vi "Puff_Dose.vi"() -> (5 "Plug in titles":string[](array[string]), 7 "Plug in values":string[](array[string]))   [LabVIEW 2022 SP3]
uses:
  Controls/Inst_type.ctl
  File/File Update Cluster.ctl
  Globals/Meas_global.vi
panel:
  in  "Show Puff Panel":bool=TRUE
  in  "Puff Stats only?":bool
  in  "Save Av puff files":bool=TRUE
  in  "Saved trace length":i32=200
  in  "Save individual puff files":bool
  in  "File Extension":string=".xls"
  in  "Save Puff Analysis file":bool
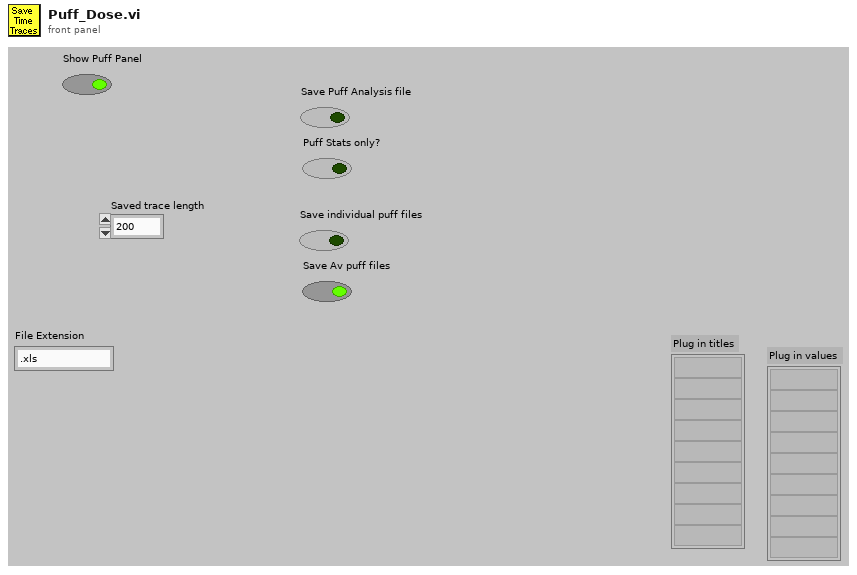
[diagram p1: front panel]
types:
  T1 = typedef "Inst_type.ctl" = enum16{"Raw voltage", "Raw with zero offsetting", "Propeller anemometer", "Pressure Transducer", "Pitot-static tube", "Hot wire", "Cross wire 1", "Cross wire 2", "Generic Linear", "Generic Polynomial", "Generic BackPoly", "Fast FID", "Thermocouple", "Cold wire", "Pulsed Wire", "LDA Vel", "LDA Tran time", "LDA Arr time", "Microphone"}
  T2 = typedef "File Update Cluster.ctl" = cluster{"File Path":path, "Rows to Add":i32[], "Extra Ch Names":string[], "Extra Ch Values":string[], "Initial Header String":string, "Separation Character":enum16{"Tab", "Comma"}}
  T3 = typedef "Analysis_info_cluster.ctl" = cluster{"Colour":u32, "Inst type":T1, "Inst name":string, "Symbol":string, "Code name":string, "Extra Info":string, "Inst Array":T4, "Extra Titles":string[], "Extra Values":string[], "U":dbl, "u^2":dbl, "u^3":dbl, "u^4":dbl, "Skew_u":dbl, "Kurt_u":dbl, "Sd Error in Mean":dbl, "% u'/U":dbl, "X":dbl, "Y":dbl, "Z":dbl, "Timescale integral Estimate":dbl, "Sd Error in Variance":dbl, "Calib File":path, "Calib Constants":dbl[], "Output Position":bool, "Stats":enum16{"None", "Basic", "Full"}, "Av Sampling Rate":dbl, "Av No of Samples":dbl, "Total Meas Time (s)":dbl, "ADAM Ch Name":string, "Max value":dbl, "Min value":dbl, "Req Sample Rate Hz":dbl, "Sync Delay Time (s)":dbl, "Ch No":i16, "Device":string, "Use Latest Calib":bool, "Port":string, "Metadata Ch Names":string[], "Metadata Ch Values":string[], "Label":string, "chState":T5, "Point Drift":dbl}
  T4 = typedef "Instrument_Array.ctl" = enum16{"PWA", "LDA", "Analogue"}
  T5 = typedef "channelState.ctl" = enum32{"No Selection", "Solo", "Mute"}
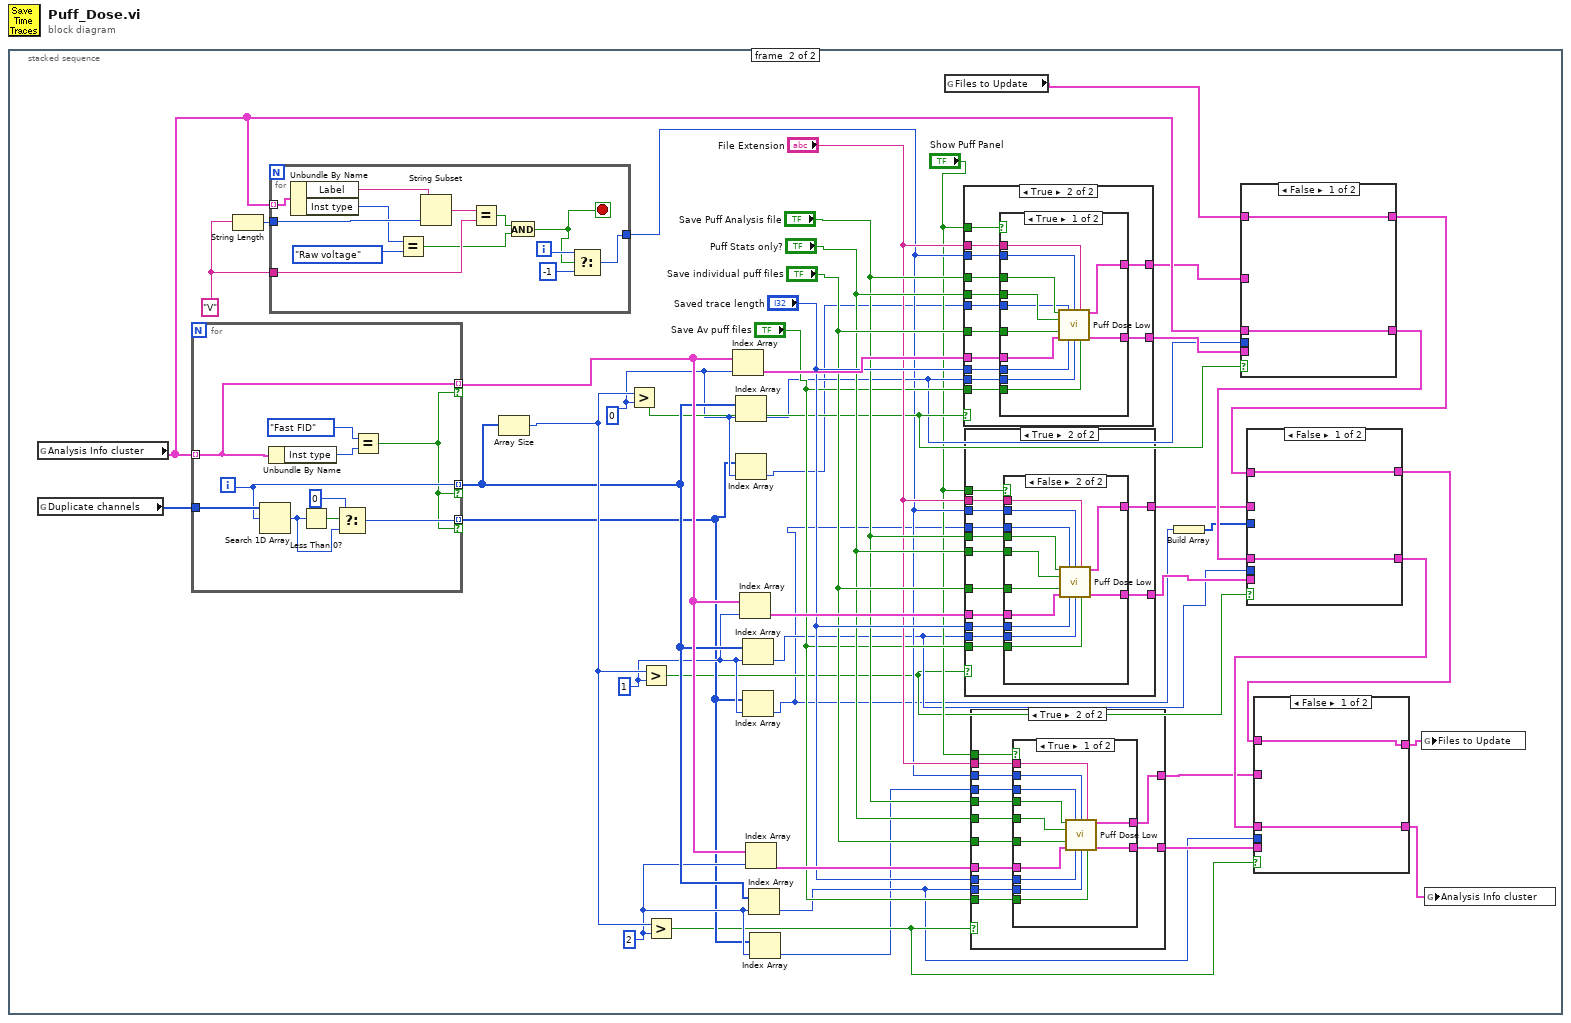
[diagram p0: block diagram]
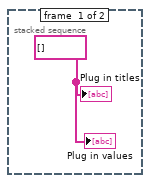
[diagram p2: hidden frame]
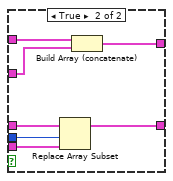
[diagram p3: hidden frame]
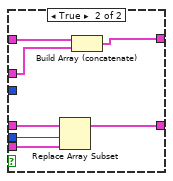
[diagram p4: hidden frame]
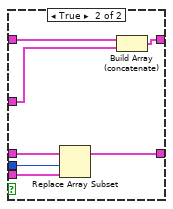
[diagram p5: hidden frame]
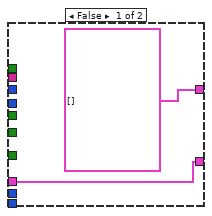
[diagram p6: hidden frame]
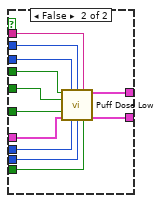
[diagram p7: hidden frame]
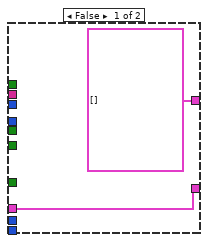
[diagram p8: hidden frame]
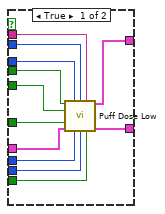
[diagram p9: hidden frame]
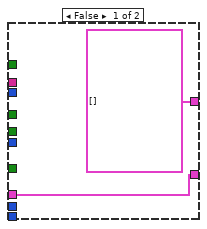
[diagram p10: hidden frame]
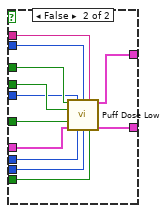
[diagram p11: hidden frame]
diagram:
  n1 = stacked-sequence {
    frame #0 {
      w1 = string[] [] ("Plug in titles")
      "Plug in titles" <- w1
      "Plug in values" <- w1
    }
    frame #1 {
      w30 = "V"
      w23 = 0 ("y")
      w25 = 2 ("y")
      w24 = 1 ("y")
      n2 = global read "Meas_global.vi" "Analysis Info cluster"() -> (w29:T3[])
      n3 = global read "Meas_global.vi" "Duplicate channels"() -> (w26:i32[])
      n4 = for {
        tunnel: w29 -> [w212] mode=indexing
        tunnel: [w212] -> w44 mode=indexing if=w205
        tunnel: [w210] -> w43 mode=indexing if=w205
        tunnel: w26 -> [w211]
        tunnel: [w206] -> w22 mode=indexing if=w205
        i -> [w210]
        n5 = Search 1D Array(1D array=w211, element=w210) -> (index of element=w208:i32)  [unwired: 1 in]
        n6 = Unbundle By Name(w212) -> ("Inst type"=w204:T1)
        n7 = Less Than 0?(x=w208) -> (x < 0?=w209:bool)
        n8 = Select(t=0, s=w209, f=w208) -> (s? t:f=w206:i32)
        n9 = Equal?(x=Inst_type."Fast FID" ("Inst type"), y=w204) -> (x = y?=w205:bool)
      }
      n10 = String Length(string=w30) -> (length=w31:i32)
      n11 = for {
        tunnel: w29 -> [w77] mode=indexing
        tunnel: [w70] -> w28
        tunnel: w31 -> [w75]
        tunnel: w30 -> [w73]
        i -> [w72]
        stop <- w65 stop-if-true
        n12 = Unbundle By Name(w77) -> ("Label"=w76:string, "Inst type"=w68:T1)
        n13 = Equal?(x=w68, y=Inst_type."Raw voltage" ("x")) -> (x = y?=w66:bool)
        n14 = String Subset(string=w76, length (rest)=w75) -> (substring=w74:string)  [unwired: 1 in]
        n15 = Equal?(x=w74, y=w73) -> (x = y?=w67:bool)
        n16 = And(x=w67, y=w66) -> (x .and. y?=w65:bool)
        n17 = Select(t=w72, s=w65, f=-1) -> (s? t:f=w70:i32)
      }
      n18 = Array Size(array=w43) -> (size(s)=w45:i32)
      n19 = Greater?(x=w45, y=w23) -> (0:w33:bool)
      n20 = Greater?(x=w45, y=w24) -> (0:w15:bool)
      n21 = Greater?(x=w45, y=w25) -> (0:w11:bool)
      n22 = Index Array(array=w44, index=w23) -> (element=w46:T3)
      n23 = Index Array(array=w43, index=w23) -> (element=w32:i32)
      n24 = Index Array(array=w22, index=w23) -> (element=w12:i32)
      n25 = Index Array(array=w44, index=w24) -> (element=w41:T3)
      n26 = Index Array(array=w43, index=w24) -> (element=w16:i32)
      n27 = Index Array(array=w22, index=w24) -> (element=w3:i32)
      n28 = Index Array(array=w44, index=w25) -> (element=w42:T3)
      n29 = Index Array(array=w43, index=w25) -> (element=w6:i32)
      n30 = Index Array(array=w22, index=w25) -> (element=w2:i32)
      n31 = global read "Meas_global.vi" "Files to Update"() -> (w20:T2[])
      n32 = case shown="True" w33 {
        tunnel: "Save Puff Analysis file" -> [_ w179]
        tunnel: "Puff Stats only?" -> [_ w178]
        tunnel: "Save individual puff files" -> [_ w177]
        tunnel: w46 -> [w166 w176]
        tunnel: "Saved trace length" -> [_ w175]
        tunnel: "Save Av puff files" -> [_ w174]
        tunnel: "File Extension" -> [_ w173]
        tunnel: w32 -> [_ w171]
        tunnel: [w166 w172] -> w34
        tunnel: w28 -> [_ w170]
        tunnel: "Show Puff Panel" -> [_ w169]
        tunnel: [T2[] [] ("File to Update") w168] -> w21
        tunnel: w12 -> [_ w167]
        frame False {
        }
        frame True {
          n33 = case shown="True" w169 {
            tunnel: w179 -> [w191 w203]
            tunnel: w178 -> [w190 w202]
            tunnel: w177 -> [w189 w201]
            tunnel: w176 -> [w188 w200]
            tunnel: w175 -> [w187 w199]
            tunnel: w174 -> [w186 w198]
            tunnel: w173 -> [w185 w197]
            tunnel: [w184 w196] -> w172
            tunnel: w171 -> [w183 w195]
            tunnel: w170 -> [w182 w194]
            tunnel: [w181 w193] -> w168
            tunnel: w167 -> [w180 w192]
            frame True {
              n34 = call "Puff Dose Low.vi"("Save Puff Analysis file"=w191, "Row Number"=w180, "Valve Index"=w182, "File Extension"=w185, "Puff Stats only?"=w190, "Save individual puff files"=w189, "Analysis info Cluster in"=w188, "Saved trace length"=w187, "FFID Index"=w183, "Save Av puff files"=w186) -> ("File to Update"=w181:T2[], "Analysis info Cluster out"=w184:T3)  [unwired: 4 in]
            }
            frame False {
              n35 = call "Puff Dose Low.vi"("Save Puff Analysis file"=w203, "Row Number"=w192, "Valve Index"=w194, "File Extension"=w197, "Puff Stats only?"=w202, "Save individual puff files"=w201, "Analysis info Cluster in"=w200, "Saved trace length"=w199, "FFID Index"=w195, "Save Av puff files"=w198) -> ("File to Update"=w193:T2[], "Analysis info Cluster out"=w196:T3)  [unwired: 4 in]
            }
          }
        }
      }
      n36 = case shown="True" w15 {
        tunnel: "Save Puff Analysis file" -> [_ w140]
        tunnel: "Puff Stats only?" -> [_ w139]
        tunnel: "Save individual puff files" -> [_ w138]
        tunnel: w41 -> [w127 w137]
        tunnel: "Saved trace length" -> [_ w136]
        tunnel: "Save Av puff files" -> [_ w135]
        tunnel: "File Extension" -> [_ w134]
        tunnel: w16 -> [_ w132]
        tunnel: [w127 w133] -> w17
        tunnel: w28 -> [_ w131]
        tunnel: "Show Puff Panel" -> [_ w130]
        tunnel: [T2[] [] ("File to Update") w129] -> w14
        tunnel: w3 -> [_ w128]
        frame False {
        }
        frame True {
          n37 = case shown="False" w130 {
            tunnel: w140 -> [w152 w164]
            tunnel: w139 -> [w151 w163]
            tunnel: w138 -> [w150 w162]
            tunnel: w137 -> [w149 w161]
            tunnel: w136 -> [w148 w160]
            tunnel: w135 -> [w147 w159]
            tunnel: w134 -> [w146 w158]
            tunnel: [w145 w157] -> w133
            tunnel: w132 -> [w144 w156]
            tunnel: w131 -> [w143 w155]
            tunnel: [w142 w154] -> w129
            tunnel: w128 -> [w141 w153]
            frame True {
              n38 = call "Puff Dose Low.vi"("Save Puff Analysis file"=w152, "Row Number"=w141, "Valve Index"=w143, "File Extension"=w146, "Puff Stats only?"=w151, "Save individual puff files"=w150, "Analysis info Cluster in"=w149, "Saved trace length"=w148, "FFID Index"=w144, "Save Av puff files"=w147) -> ("File to Update"=w142:T2[], "Analysis info Cluster out"=w145:T3)  [unwired: 4 in]
            }
            frame False {
              n39 = call "Puff Dose Low.vi"("Save Puff Analysis file"=w164, "Row Number"=w153, "Valve Index"=w155, "File Extension"=w158, "Puff Stats only?"=w163, "Save individual puff files"=w162, "Analysis info Cluster in"=w161, "Saved trace length"=w160, "FFID Index"=w156, "Save Av puff files"=w159) -> ("File to Update"=w154:T2[], "Analysis info Cluster out"=w157:T3)  [unwired: 4 in]
            }
          }
        }
      }
      n40 = case shown="True" w11 {
        tunnel: "Save Puff Analysis file" -> [_ w101]
        tunnel: "Puff Stats only?" -> [_ w100]
        tunnel: "Save individual puff files" -> [_ w99]
        tunnel: w42 -> [w88 w98]
        tunnel: "Saved trace length" -> [_ w97]
        tunnel: "Save Av puff files" -> [_ w96]
        tunnel: "File Extension" -> [_ w95]
        tunnel: w6 -> [_ w94]
        tunnel: [w88 w93] -> w7
        tunnel: w28 -> [_ w92]
        tunnel: "Show Puff Panel" -> [_ w91]
        tunnel: [T2[] [] ("File to Update") w90] -> w5
        tunnel: w2 -> [_ w89]
        frame False {
        }
        frame True {
          n41 = case shown="True" w91 {
            tunnel: w101 -> [w113 w125]
            tunnel: w100 -> [w112 w124]
            tunnel: w99 -> [w111 w123]
            tunnel: w98 -> [w110 w122]
            tunnel: w97 -> [w109 w121]
            tunnel: w96 -> [w108 w120]
            tunnel: w95 -> [w107 w119]
            tunnel: w94 -> [w106 w118]
            tunnel: [w105 w117] -> w93
            tunnel: w92 -> [w104 w116]
            tunnel: [w103 w115] -> w90
            tunnel: w89 -> [w102 w114]
            frame True {
              n42 = call "Puff Dose Low.vi"("Save Puff Analysis file"=w113, "Row Number"=w102, "Valve Index"=w104, "File Extension"=w107, "Puff Stats only?"=w112, "Save individual puff files"=w111, "Analysis info Cluster in"=w110, "Saved trace length"=w109, "FFID Index"=w106, "Save Av puff files"=w108) -> ("File to Update"=w103:T2[], "Analysis info Cluster out"=w105:T3)  [unwired: 4 in]
            }
            frame False {
              n43 = call "Puff Dose Low.vi"("Save Puff Analysis file"=w125, "Row Number"=w114, "Valve Index"=w116, "File Extension"=w119, "Puff Stats only?"=w124, "Save individual puff files"=w123, "Analysis info Cluster in"=w122, "Saved trace length"=w121, "FFID Index"=w118, "Save Av puff files"=w120) -> ("File to Update"=w115:T2[], "Analysis info Cluster out"=w117:T3)  [unwired: 4 in]
            }
          }
        }
      }
      n44 = Build Array(w3) -> (w13:i32[])
      n45 = case shown="False" w33 {
        tunnel: w29 -> [w79 w86]
        tunnel: w34 -> [_ w85]
        tunnel: w32 -> [_ w84]
        tunnel: [w79 w83] -> w19
        tunnel: w21 -> [_ w80]
        tunnel: w20 -> [w78 w82]
        tunnel: [w78 w81] -> w18
        frame False {
        }
        frame True {
          n46 = Replace Array Subset(array=w86, new element=w85, index=w84) -> (w83:T3[])
          n47 = Build Array (concatenate)(w82, w80) -> (w81:T2[])
        }
      }
      n48 = case shown="False" w15 {
        tunnel: w19 -> [w57 w64]
        tunnel: w17 -> [_ w63]
        tunnel: w16 -> [_ w62]
        tunnel: [w57 w61] -> w9
        tunnel: w14 -> [_ w59]
        tunnel: w13 -> [_ _]
        tunnel: w18 -> [w56 w60]
        tunnel: [w56 w58] -> w10
        frame False {
        }
        frame True {
          n49 = Replace Array Subset(array=w64, new element=w63, index=w62) -> (w61:T3[])
          n50 = Build Array (concatenate)(w60, w59) -> (w58:T2[])
        }
      }
      n51 = case shown="False" w11 {
        tunnel: w9 -> [w48 w55]
        tunnel: w7 -> [_ w54]
        tunnel: w6 -> [_ w53]
        tunnel: [w48 w52] -> w8
        tunnel: w5 -> [_ w50]
        tunnel: w10 -> [w47 w51]
        tunnel: [w47 w49] -> w4
        frame False {
        }
        frame True {
          n52 = Replace Array Subset(array=w55, new element=w54, index=w53) -> (w52:T3[])
          n53 = Build Array (concatenate)(w51, w50) -> (w49:T2[])
        }
      }
      n54 = global write "Meas_global.vi" "Files to Update"(w4) -> ()
      n55 = global write "Meas_global.vi" "Analysis Info cluster"(w8) -> ()
    }
  }
